vi "Export - Rx Packet.vi"(8 "error in (no error)":errorcluster, 11 "Device Item Ref in":T10 format="%.0x") -> (0 "error out":errorcluster, 3 "Rx Packet":T1 {"targetPriority" min=-2 max=16 step=1; "targetProcessor" min=-2 max=16 step=1; "Endianness" items=["big-endian"=0, "little-endian"=2]})   [LabVIEW 2019, in "UDP-Custom-Device System Explorer.lvlib"]
uses:
  UDP-Custom-Device System Explorer.lvlib
  <vilib>/NI VeriStand/Custom Device API/Custom Device Item Ref.ctl
  Types/XML - New/ImpExp - Rx Packet Data.ctl
  <vilib>/NI VeriStand/Custom Device API/Custom Device Item Info.ctl
  Shared/Types/Shared - Channel Data Type.ctl
  Shared/Types/Shared - Buffered.PacketInfo.ctl
  Shared/Types/Shared - Pointer Encoding.ctl
  Shared/Types/Shared - Receive Buffer Options.ctl
  Shared/Types/Shared - Transmit Buffer Options.ctl
  Shared/Types/Shared - New Data Options.ctl
  Shared/Types/Shared - Thread Management.ctl
  Property Accessors/Shared Packet Accessors.lvlib
  <vilib>/NI VeriStand/Custom Device API/Custom Device API.lvlib
  Property Accessors/Rx Packet Accessors.lvlib
  Shared/UDP-Custom-Device Shared.lvlib
  Property Accessors/Rx Channel Accessors.lvlib
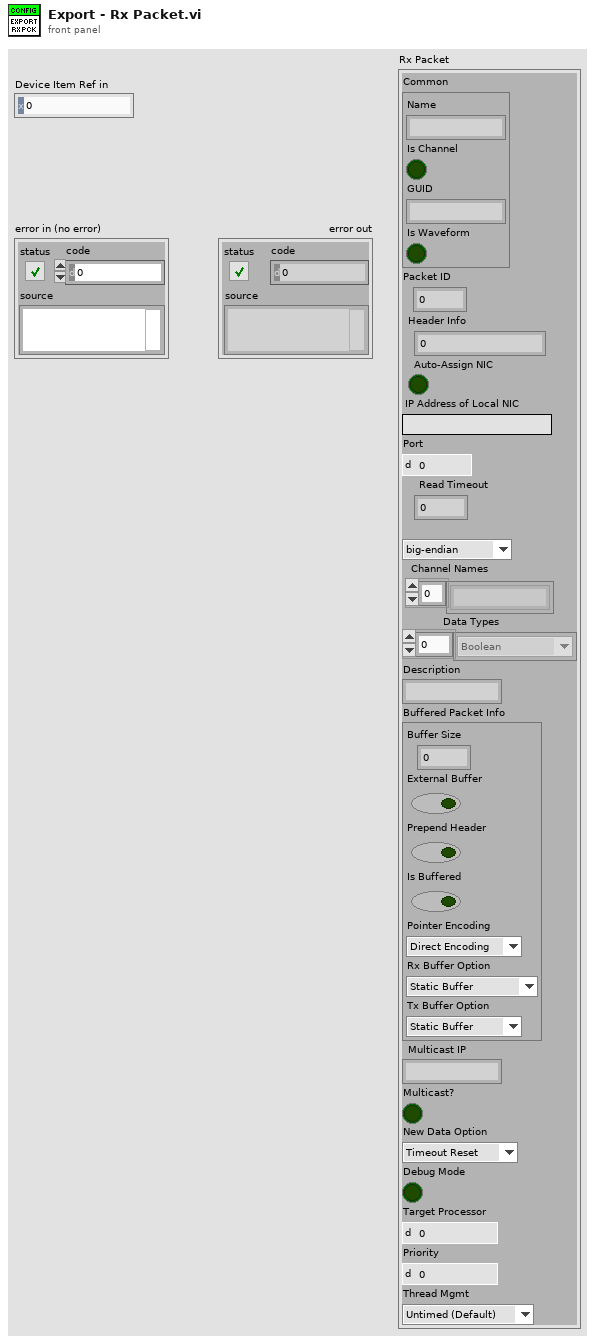
[diagram p1: front panel]
types:
  T1 = typedef "UDP-Custom-Device System Explorer.lvlib/ImpExp - Rx Packet Data.ctl" = cluster{"Common":T2, "Packet ID":i32, "Header Info":u32, "Auto-Assign NIC":bool, "IP Address of Local NIC":string, "Port":u16, "Read Timeout":i32, "Endianness":u16, "Channel Names":string[], "Data Types":T3[], "Description":string, "Buffered Packet Info":T4, "Multicast IP":string, "Multicast?":bool, "New Data Option":T8, "Debug Mode":bool, "targetProcessor":i8, "targetPriority":i16, "Thread Mgmt":T9}
  T2 = typedef "Custom Device API.lvlib/Custom Device Item Info.ctl" = cluster{"Name":string, "Is Channel":bool, "GUID":string, "Is Waveform":bool}
  T3 = typedef "UDP-Custom-Device Shared.lvlib/Shared - Channel Data Type.ctl" = enum16{"Boolean", "Single", "Double", "I8", "I16", "I32", "I64", "U8", "U16", "U32", "U64"}
  T4 = typedef "UDP-Custom-Device Shared.lvlib/Shared - Buffered.PacketInfo.ctl" = cluster{"Buffer Size":i32, "External Buffer":bool, "Prepend Header":bool, "Is Buffered":bool, "Pointer Encoding":T5, "Rx Buffer Option":T6, "Tx Buffer Option":T7}
  T5 = typedef "UDP-Custom-Device Shared.lvlib/Shared - Pointer Encoding.ctl" = enum16{"Direct Encoding", "Conversion Encoding"}
  T6 = typedef "UDP-Custom-Device Shared.lvlib/Shared - Receive Buffer Options.ctl" = enum16{"Static Buffer", "Circular Buffer", "Circular Buffer + Size", "Internal Cache", "Internal Cache + Size", "Ping Pong", "Ping Pong + Size"}
  T7 = typedef "UDP-Custom-Device Shared.lvlib/Shared - Transmit Buffer Options.ctl" = enum16{"Static Buffer", "FIFO Buffer", "FIFO Buffer + Port"}
  T8 = typedef "UDP-Custom-Device Shared.lvlib/Shared - New Data Options.ctl" = enum16{"Timeout Reset", "Counter"}
  T9 = typedef "UDP-Custom-Device Shared.lvlib/Shared - Thread Management.ctl" = enum16{"Untimed (Default)", "Timed (High Priority)"}
  T10 = typedef "Custom Device API.lvlib/Custom Device Item Ref.ctl" = u64
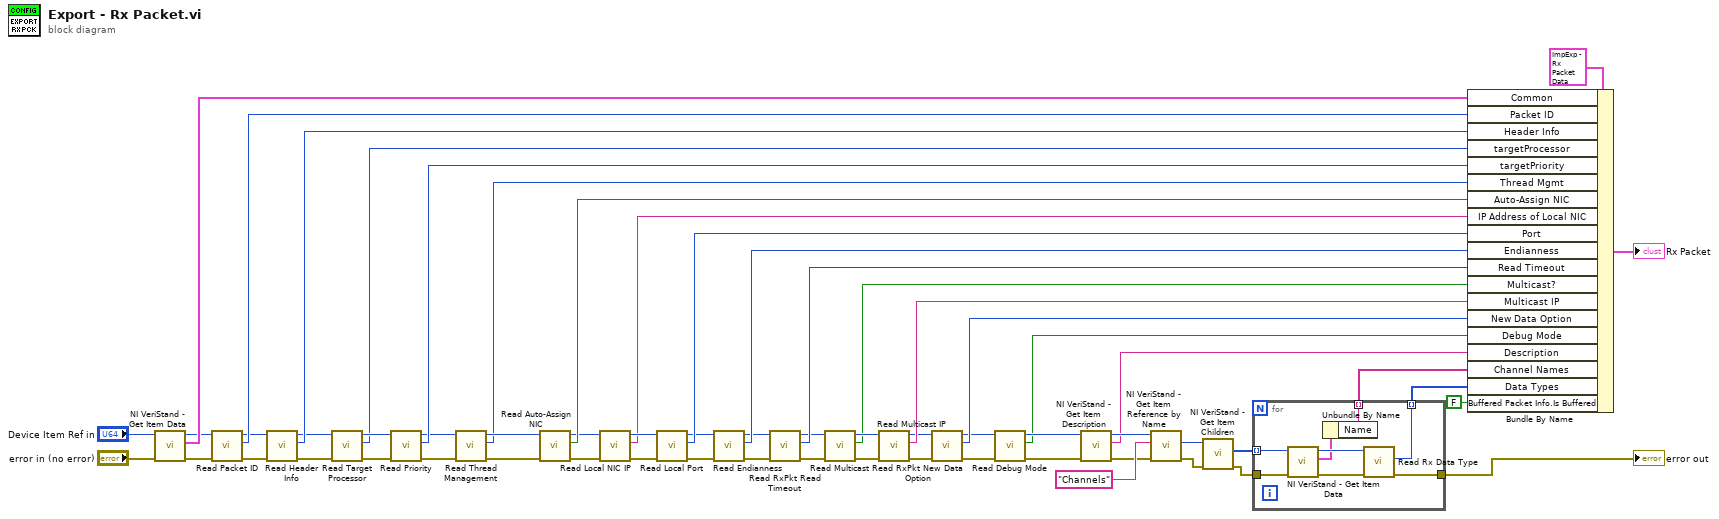
[diagram p0: block diagram]
diagram:
  n1 = call <vilib>:"NI VeriStand - Get Item Data.vi"("error in (no error)"="error in (no error)", "Item Ref in"="Device Item Ref in") -> ("error out"=w44:errorcluster, "Item Info"=w58:T2, "Item Ref out"=w57:T10)  [unwired: 6 in, 1 out]
  n2 = call "Read Packet ID.vi"("error in (no error)"=w44, "Node Ptr"=w57) -> ("error out"=w54:errorcluster, "Packet ID"=w56:i32, "Node Ptr out"=w55:T10)  [unwired: 7 in]
  n3 = call "Read Header Info.vi"("error in (no error)"=w54, "Node Ptr"=w55) -> ("error out"=w8:errorcluster, "Header Info"=w53:u32, "Node Ptr out"=w9:T10)  [unwired: 7 in]
  n4 = call "Read Target Processor.vi"("error in (no error)"=w8, "Node Ptr"=w9) -> ("error out"=w10:errorcluster, "targetProcessor"=w7:i8, "Node Ptr out"=w11:T10)  [unwired: 7 in]
  n5 = call "Read Priority.vi"("error in (no error)"=w10, "Node Ptr"=w11) -> ("error out"=w5:errorcluster, "targetPriority"=w6:i16, "Node Ptr out"=w3:T10)  [unwired: 7 in]
  n6 = call "Read Thread Management.vi"("error in (no error)"=w5, "Node Ptr"=w3) -> ("error out"=w4:errorcluster, "Thread Management"=w1:T9, "Node Ptr out"=w2:T10)  [unwired: 7 in]
  n7 = call "Read Auto-Assign NIC.vi"("error in (no error)"=w4, "Node Ptr"=w2) -> ("error out"=w48:errorcluster, "Auto-Assign NIC"=w52:bool, "Node Ptr out"=w51:T10)  [unwired: 7 in]
  n8 = call "Read Local NIC IP.vi"("error in (no error)"=w48, "Node Ptr"=w51) -> ("error out"=w49:errorcluster, "IP Address of Local NIC"=w47:string, "Node Ptr out"=w50:T10)  [unwired: 7 in]
  n9 = call "Read Local Port.vi"("error in (no error)"=w49, "Node Ptr"=w50) -> ("error out"=w42:errorcluster, "Port"=w46:u16, "Node Ptr out"=w41:T10)  [unwired: 7 in]
  n10 = call "Read Endianness.vi"("error in (no error)"=w42, "Node Ptr"=w41) -> ("error out"=w39:errorcluster, "Endianness"=w45:u16, "Node Ptr out"=w38:T10)  [unwired: 7 in]
  n11 = call "Read RxPkt Read Timeout.vi"("error in (no error)"=w39, "Node Ptr"=w38) -> ("error out"=w20:errorcluster, "Read Timeout"=w40:i32, "Node Ptr out"=w21:T10)  [unwired: 7 in]
  n12 = call "Read Multicast.vi"("error in (no error)"=w20, "Node Ptr"=w21) -> ("error out"=w24:errorcluster, "Multicast"=w23:bool, "Node Ptr out"=w25:T10)  [unwired: 7 in]
  n13 = call "Read Multicast IP.vi"("error in (no error)"=w24, "Node Ptr"=w25) -> ("error out"=w18:errorcluster, "Multicast IP Address"=w22:string, "Node Ptr out"=w19:T10)  [unwired: 7 in]
  n14 = call "Read RxPkt New Data Option.vi"("error in (no error)"=w18, "Node Ptr"=w19) -> ("error out"=w14:errorcluster, "New Data Option"=w17:T8, "Node Ptr out"=w16:T10)  [unwired: 7 in]
  n15 = call "Read Debug Mode.vi"("error in (no error)"=w14, "Node Ptr"=w16) -> ("error out"=w13:errorcluster, "Debug Mode"=w12:bool, "Node Ptr out"=w15:T10)  [unwired: 7 in]
  n16 = call <vilib>:"NI VeriStand - Get Item Description.vi"("error in (no error)"=w13, "Item Ref in"=w15) -> ("error out"=w29:errorcluster, "Description"=w27:string, "Item Ref out"=w28:T10)  [unwired: 6 in, 1 out]
  n17 = call <vilib>:"NI VeriStand - Get Item Reference by Name.vi"("error in (no error)"=w29, "Item Name"="Channels" ("Section Name"), "Parent Ref in"=w28) -> ("error out"=w35:errorcluster, "Item Ref"=w36:T10)  [unwired: 5 in, 2 out]
  n18 = call <vilib>:"NI VeriStand - Get Item Children.vi"("error in (no error)"=w35, "Item Ref in"=w36) -> ("error out"=w33:errorcluster, "Child Refs"=w34:T10[])  [unwired: 6 in, 2 out]
  n19 = for {
    tunnel: w34 -> [w69] mode=indexing
    tunnel: w33 -> [w67]
    tunnel: [w65] -> w32
    tunnel: [w63] -> w31 mode=indexing
    tunnel: [w62] -> w30 mode=indexing
    n20 = call <vilib>:"NI VeriStand - Get Item Data.vi"("error in (no error)"=w67, "Item Ref in"=w69) -> ("error out"=w66:errorcluster, "Item Info"=w64:T2, "Item Ref out"=w68:T10)  [unwired: 6 in, 1 out]
    n21 = Unbundle By Name(w64) -> ("Name"=w63:string)
    n22 = call "Read Rx Data Type.vi"("error in (no error)"=w66, "Node Ptr"=w68) -> ("error out"=w65:errorcluster, "Data Type"=w62:T3)  [unwired: 7 in, 1 out]
  }
  "error out" <- w32
  n23 = Bundle By Name(cluster=T1 {"Common"={"Name"="", "Is Channel"=FALSE, "GUID"="", "Is Waveform"=FALSE}, "Packet ID"=0, "Header Info"=0, "Auto-Assign NIC"=FALSE, "IP Address of Local NIC"="", "Port"=0, "Read Timeout"=0, "Endianness"=0, "Channel Names"=[], "Data Types"=[], "Description"="", "Buffered Packet Info"={"Buffer Size"=0, "External Buffer"=FALSE, "Prepend Header"=FALSE, "Is Buffered"=FALSE, "Pointer Encoding"=enum."Direct Encoding", "Rx Buffer Option"=enum."Static Buffer", "Tx Buffer Option"=enum."Static Buffer"}, "Multicast IP"="", "Multicast?"=FALSE, "New Data Option"=enum."Timeout Reset", "Debug Mode"=FALSE, "targetProcessor"=0, "targetPriority"=0, "Thread Mgmt"=enum."Untimed (Default)"} ("Rx Packet"), "Common"=w58, "Packet ID"=w56, "Header Info"=w53, "targetProcessor"=w7, "targetPriority"=w6, "Thread Mgmt"=w1, "Auto-Assign NIC"=w52, "IP Address of Local NIC"=w47, "Port"=w46, "Endianness"=w45, "Read Timeout"=w40, "Multicast?"=w23, "Multicast IP"=w22, "New Data Option"=w17, "Debug Mode"=w12, "Description"=w27, "Channel Names"=w31, "Data Types"=w30, "Buffered Packet Info.Is Buffered"=FALSE) -> (→"Rx Packet":T1)
